vi "Linear_Flow_Ramp.vi"(2 "Debug Mode":bool, 3 "Elapsed Time (s)":dbl, 4 "State":enum16{"Edit", "Start", "Run", "End", "Idle"}(ring), 5 "Argument List In":string[](array[string])) -> (0 "Status Out":string, 1 "Argument List Out":string[](array[string]))   [LabVIEW 2011]
panel:
  in  "Flow to Ramp":u16(ring) items=["Flow1"]
  in  "Select":enum32{"Use Time/End Flow", "Use Rate"}(radio)
  in  "End Flow":dbl caption="End Flow\n(sccm)"
  in  "Total Time":dbl caption="Total Time (sec)"
  in  "Ramp Rate":dbl caption="Ramp Rate\n(sccm/sec)"
  in  "Start Flow":dbl caption="Start Flow\n(sccm)"
  in  "Gas":u16(ring)=5 items=["R_Al", "R_As_Liq", "R_AsH3", "R_Fe", "R_Ga", "R_H2", "R_In", "R_N_Dop", "R_N2", "R_P_Dop", "R_P_Liq", "R_PH3"]
  in  "Run":bool
  in  "Gas Source In":bool
  in  "H2 Flush":bool
  in  "Bubbler In":bool
  in  "H2 Dilute":bool
  in  "Cancel":bool
  in  "OK":bool
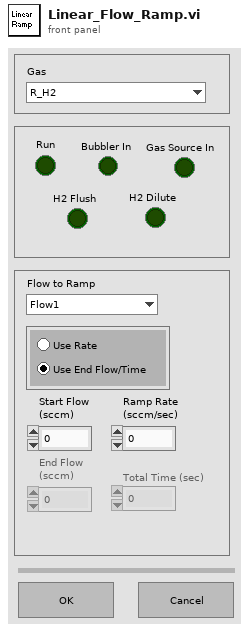
[diagram p1: front panel]
types:
  T1 = enum16{"Discrete", "Continuous", "Instantaneous"}
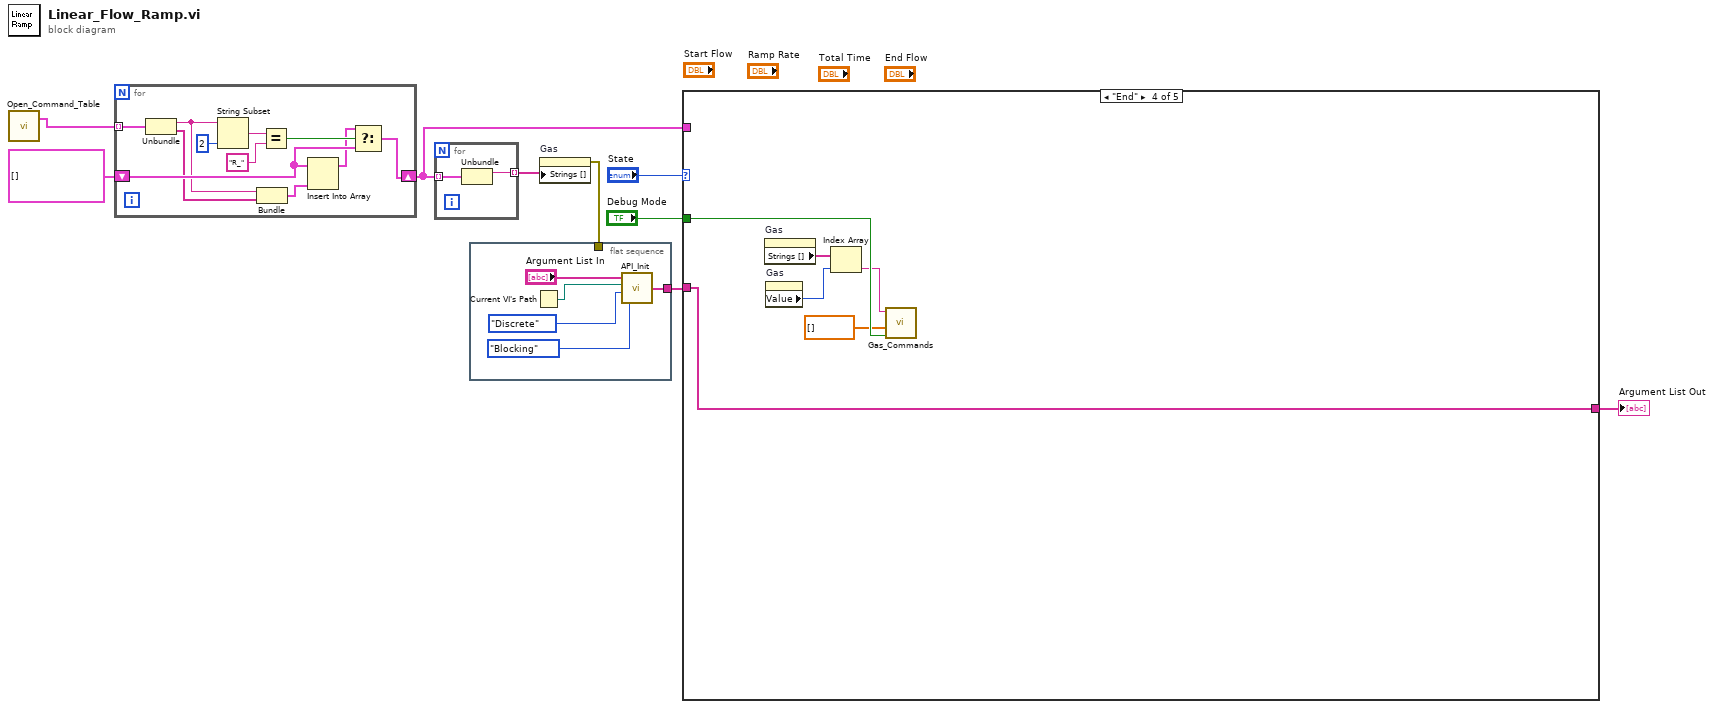
[diagram p0: block diagram]
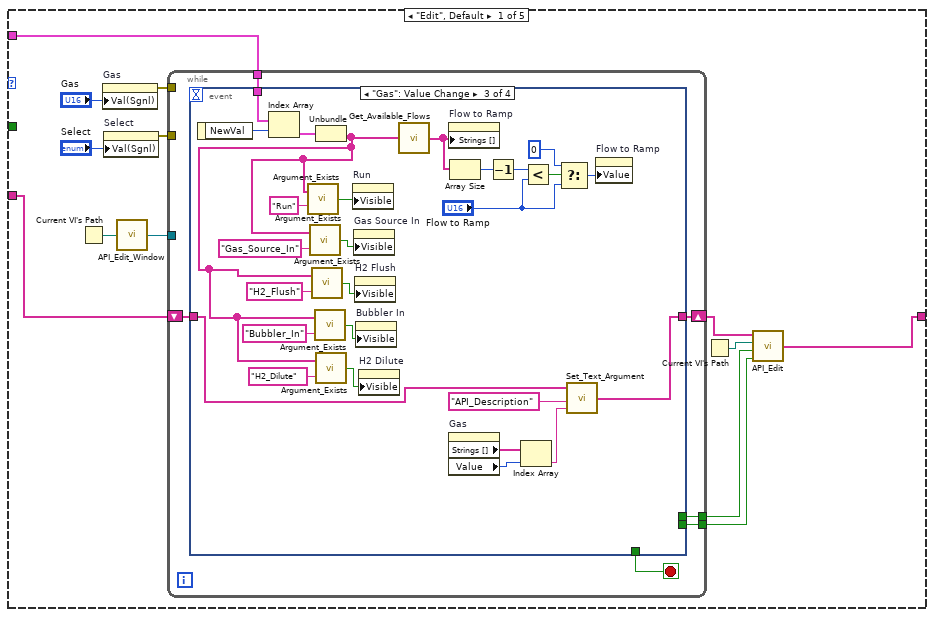
[diagram p2: hidden frame]
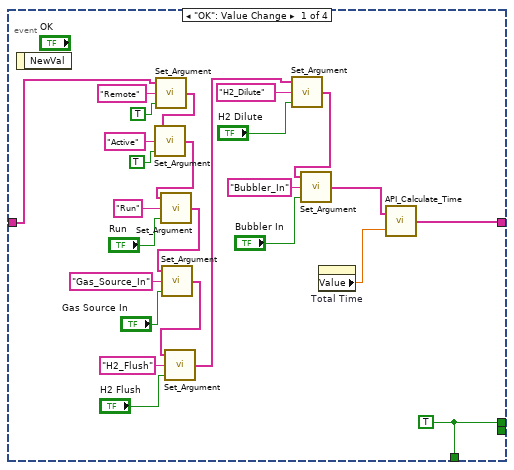
[diagram p3: hidden frame]
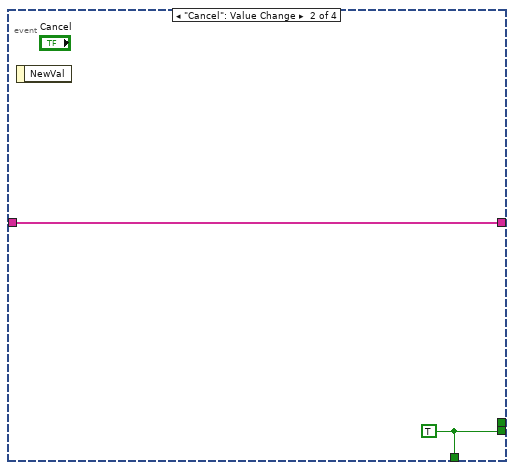
[diagram p4: hidden frame]
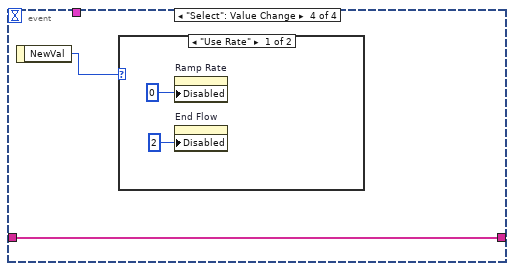
[diagram p5: hidden frame]
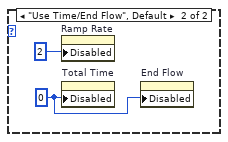
[diagram p6: hidden frame]
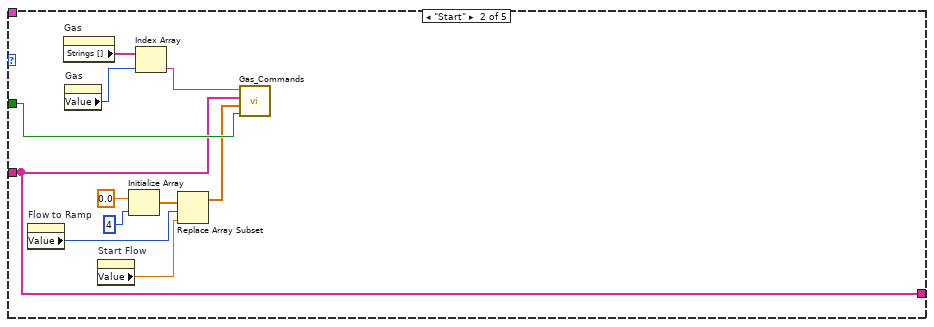
[diagram p7: hidden frame]
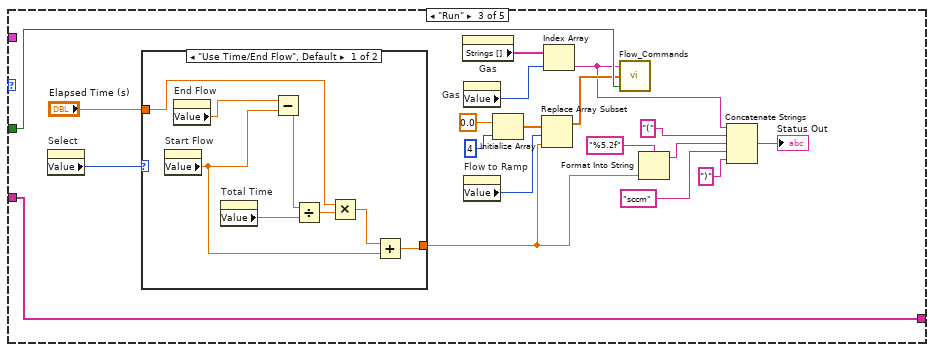
[diagram p8: hidden frame]
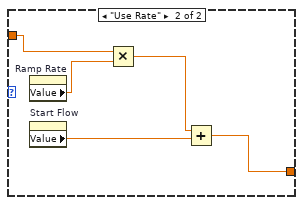
[diagram p9: hidden frame]
diagram:
  n1 = call "Open_Command_Table.vi"() -> ("Commands"=w3:cluster{string, string[]}[])  [unwired: 2 out]
  n2 = for {
    tunnel: w3 -> [w20] mode=indexing
    shift-right: [w15] -> w2
    shift-left: cluster{string, string[]}[] [] ("Commands") -> [w14]
    n3 = Unbundle(w20) -> (w12:string, w11:string[])
    n4 = String Subset(string=w12, length (rest)=2 ("length (rest)")) -> (substring=w18:string)  [unwired: 1 out]
    n5 = Bundle(w12, w11) -> (w10:cluster{string, string[]})  [unwired: 1 out]
    n6 = Equal?(x=w18, y="R_") -> (x = y?=w16:bool)
    n7 = Insert Into Array(array=w14, new element=w10) -> (w13:cluster{string, string[]}[])  [unwired: 1 in]
    n8 = Select(t=w13, s=w16, f=w14) -> (s? t:f=w15:cluster{string, string[]}[])
  }
  n9 = for {
    tunnel: w2 -> [w22] mode=indexing
    tunnel: [w21] -> w5 mode=indexing
    n10 = Unbundle(w22) -> (w21:string)  [unwired: 1 out]
  }
  n11 = flat-sequence {
    tunnel: [w27] -> w6
    tunnel: w1 -> [_]
    frame #0 {
      n12 = Current VI's Path() -> (path=w24:path)
      n13 = call "API_Init.vi"("API Option"=enum16{"None", "Blocking", "Wait for Input"}."Blocking", "API Mode"=T1."Discrete", "VI Path"=w24, "Argument List In"="Argument List In") -> ("Argument List Out"=w27:string[])
    }
  }
  n14 = property on="Gas" class="Ring (strict)"("Strings []"=w5) -> (error out=w1:errorcluster)  [unwired: 2 in, 1 out]
  n15 = case shown="\"End\"" "State" {
    tunnel: [w30 w110 w121 w153 w156] -> w8
    tunnel: w6 -> [w31 w110 w121 w153 w156]
    tunnel: "Debug Mode" -> [_ w117 w136 w155 _]
    tunnel: w2 -> [w34 _ _ _ _]
    frame "Edit", Default {
      n16 = Current VI's Path() -> (path=w36:path)
      n17 = property on="Gas" class="Ring (strict)"("Val(Sgnl)"="Gas") -> (error out=w32:errorcluster)  [unwired: 2 in, 1 out]
      n18 = property on="Select" class="RadioBtnsControl (strict)"("Val(Sgnl)"="Select") -> (error out=w28:errorcluster)  [unwired: 2 in, 1 out]
      n19 = call "API_Edit_Window.vi"("VI Path"=w36) -> ("VI Reference"=w35:refnum<vi>)
      n20 = while {
        tunnel: w34 -> [w45]
        tunnel: [w43] -> w38
        tunnel: [w42] -> w37
        tunnel: w35 -> [_]
        tunnel: w32 -> [_]
        shift-right: [w46] -> w39
        shift-left: w31 -> [w41]
        tunnel: w28 -> [_]
        stop <- w44 stop-if-true
        n21 = event shown="[2] \"Gas\": Value Change" {
          selector: _ -> [_ _ _ _]
          dyn-events: _ -> [_ _ _ _]
          timeout: _ -> [_ _ _ _]
          tunnel: w41 -> [w70 w73 w74 w101]
          tunnel: [w47 w73 w79 w101] -> w46
          tunnel: w45 -> [_ _ w100 _]
          tunnel: [w71 w72 _ _] -> w44
          tunnel: [w71 _ _ _] -> w43
          tunnel: [_ w72 _ _] -> w42
          event "OK": Value Change {
            w71 = TRUE
            n22 = event-data() -> ()  [unwired: 2 out]
            n23 = call "Set_Argument.vi"("Enable"=TRUE, "Argument"="Remote", "Argument List In"=w70) -> ("Argument List Out"=w51:string[])
            n24 = call "Set_Argument.vi"("Enable"=TRUE, "Argument"="Active", "Argument List In"=w51) -> ("Argument List Out"=w50:string[])
            n25 = call "Set_Argument.vi"("Enable"="Run", "Argument"="Run", "Argument List In"=w50) -> ("Argument List Out"=w65:string[])
            n26 = call "Set_Argument.vi"("Enable"="Gas Source In", "Argument"="Gas_Source_In", "Argument List In"=w65) -> ("Argument List Out"=w62:string[])
            n27 = call "Set_Argument.vi"("Enable"="H2 Flush", "Argument"="H2_Flush", "Argument List In"=w62) -> ("Argument List Out"=w59:string[])
            n28 = call "Set_Argument.vi"("Enable"="H2 Dilute", "Argument"="H2_Dilute", "Argument List In"=w59) -> ("Argument List Out"=w56:string[])
            n29 = call "Set_Argument.vi"("Enable"="Bubbler In", "Argument"="Bubbler_In", "Argument List In"=w56) -> ("Argument List Out"=w48:string[])
            n30 = property on="Total Time" class="DigNum (strict)"() -> ("Value"=w49:dbl)  [unwired: 2 in, 2 out]
            n31 = call "API_Calculate_Time.vi"("Time"=w49, "Argument List In"=w48) -> ("Argument List Out"=w47:string[])
          }
          event "Cancel": Value Change {
            w72 = TRUE
            n32 = event-data() -> ()  [unwired: 2 out]
          }
          event "Gas": Value Change {
            n33 = event-data() -> ("NewVal"=w88:u16)  [unwired: 1 out]
            n34 = Index Array(array=w100, index=w88) -> (element=w99:cluster{string, string[]})
            n35 = Unbundle(w99) -> (w83:string[])  [unwired: 1 out]
            n36 = call "Argument_Exists.vi"("Argument"="Run", "Argument List"=w83) -> ("Argument Exists"=w97:bool)
            n37 = call "Argument_Exists.vi"("Argument"="Gas_Source_In", "Argument List"=w83) -> ("Argument Exists"=w93:bool)
            n38 = call "Argument_Exists.vi"("Argument"="H2_Flush", "Argument List"=w83) -> ("Argument Exists"=w94:bool)
            n39 = call "Argument_Exists.vi"("Argument"="Bubbler_In", "Argument List"=w83) -> ("Argument Exists"=w91:bool)
            n40 = call "Argument_Exists.vi"("Argument"="H2_Dilute", "Argument List"=w83) -> ("Argument Exists"=w89:bool)
            n41 = property on="Run" class="Bool (strict)"("Visible"=w97) -> ()  [unwired: 2 in, 2 out]
            n42 = property on="Gas Source In" class="Bool (strict)"("Visible"=w93) -> ()  [unwired: 2 in, 2 out]
            n43 = property on="H2 Flush" class="Bool (strict)"("Visible"=w94) -> ()  [unwired: 2 in, 2 out]
            n44 = property on="Bubbler In" class="Bool (strict)"("Visible"=w91) -> ()  [unwired: 2 in, 2 out]
            n45 = property on="H2 Dilute" class="Bool (strict)"("Visible"=w89) -> ()  [unwired: 2 in, 2 out]
            n46 = call "Get_Available_Flows.vi"("Argument List"=w83) -> ("Available Flows"=w81:string[])
            n47 = property on="Flow to Ramp" class="Ring (strict)"("Strings []"=w81) -> ()  [unwired: 2 in, 2 out]
            n48 = property on="Gas" class="Ring (strict)"() -> ("Strings []"=w78:string[], "Value"=w77:u16)  [unwired: 2 in, 2 out]
            n49 = Array Size(array=w81) -> (size(s)=w87:i32)
            n50 = Decrement(x=w87) -> (x-1=w85:i32)
            n51 = Index Array(array=w78, index=w77) -> (element=w76:string)
            n52 = Less?(x=w85, y="Flow to Ramp") -> (x < y?=w86:bool)
            n53 = Select(t=u16 0, s=w86, f="Flow to Ramp") -> (s? t:f=w75:u16)
            n54 = call "Set_Text_Argument.vi"("Text"=w76, "Argument"="API_Description", "Argument List In"=w74) -> ("Argument List Out"=w79:string[])
            n55 = property on="Flow to Ramp" class="Ring (strict)"("Value"=w75) -> ()  [unwired: 2 in, 2 out]
          }
          event "Select": Value Change {
            n56 = event-data() -> ("NewVal"=w102:enum32{"Use Time/End Flow", "Use Rate"})  [unwired: 1 out]
            n57 = case shown="\"Use Rate\"" w102 {
              frame "Use Rate" {
                n58 = property on="Ramp Rate" class="DigNum (strict)"("Disabled"=u8 0) -> ()  [unwired: 2 in, 2 out]
                n59 = property on="End Flow" class="DigNum (strict)"("Disabled"=u8 2) -> ()  [unwired: 2 in, 2 out]
              }
              frame "Use Time/End Flow", Default {
                w105 = u8 0 ("Disabled")
                n60 = property on="Ramp Rate" class="DigNum (strict)"("Disabled"=u8 2) -> ()  [unwired: 2 in, 2 out]
                n61 = property on="Total Time" class="DigNum (strict)"("Disabled"=w105) -> ()  [unwired: 2 in, 2 out]
                n62 = property on="End Flow" class="DigNum (strict)"("Disabled"=w105) -> ()  [unwired: 2 in, 2 out]
              }
            }
          }
        }
      }
      n63 = Current VI's Path() -> (path=w40:path)
      n64 = call "API_Edit.vi"("Cancel"=w37, "OK"=w38, "VI Path"=w40, "Argument List In"=w39) -> ("Argument List Out"=w30:string[])
    }
    frame "Start" {
      n65 = property on="Flow to Ramp" class="Ring (strict)"() -> ("Value"=w114:u16)  [unwired: 2 in, 2 out]
      n66 = property on="Gas" class="Ring (strict)"() -> ("Strings []"=w109:string[])  [unwired: 2 in, 2 out]
      n67 = property on="Gas" class="Ring (strict)"() -> ("Value"=w108:u16)  [unwired: 2 in, 2 out]
      n68 = property on="Start Flow" class="DigNum (strict)"() -> ("Value"=w112:dbl)  [unwired: 2 in, 2 out]
      n69 = Initialize Array(0.0 ("element"), 4 ("dimension size")) -> (w113:dbl[])
      n70 = Index Array(array=w109, index=w108) -> (element=w107:string)
      n71 = Replace Array Subset(array=w113, new element=w112, index=w114) -> (w111:dbl[])
      n72 = call "Gas_Commands.vi"("Debug Mode"=w117, "Flow Array"=w111, "Argument List"=w110, "Command"=w107) -> ()  [unwired: 1 out]
    }
    frame "Run" {
      n73 = property on="Select" class="RadioBtnsControl (strict)"() -> ("Value"=w122:enum32{"Use Time/End Flow", "Use Rate"})  [unwired: 2 in, 2 out]
      n74 = case shown="\"Use Time/End Flow\", Default" w122 {
        tunnel: "Elapsed Time (s)" -> [w143 w149]
        tunnel: [w137 w145] -> w126
        frame "Use Time/End Flow", Default {
          n75 = property on="Start Flow" class="DigNum (strict)"() -> ("Value"=w139:dbl)  [unwired: 2 in, 2 out]
          n76 = property on="End Flow" class="DigNum (strict)"() -> ("Value"=w141:dbl)  [unwired: 2 in, 2 out]
          n77 = property on="Total Time" class="DigNum (strict)"() -> ("Value"=w142:dbl)  [unwired: 2 in, 2 out]
          n78 = Subtract(x=w141, y=w139) -> (x-y=w140:dbl)
          n79 = Divide(x=w140, y=w142) -> (x/y=w144:dbl)
          n80 = Multiply(x=w143, y=w144) -> (x*y=w138:dbl)
          n81 = Add(x=w138, y=w139) -> (x+y=w137:dbl)
        }
        frame "Use Rate" {
          n82 = property on="Ramp Rate" class="DigNum (strict)"() -> ("Value"=w148:dbl)  [unwired: 2 in, 2 out]
          n83 = property on="Start Flow" class="DigNum (strict)"() -> ("Value"=w146:dbl)  [unwired: 2 in, 2 out]
          n84 = Multiply(x=w149, y=w148) -> (x*y=w147:dbl)
          n85 = Add(x=w147, y=w146) -> (x+y=w145:dbl)
        }
      }
      n86 = property on="Gas" class="Ring (strict)"() -> ("Strings []"=w119:string[])  [unwired: 2 in, 2 out]
      n87 = property on="Gas" class="Ring (strict)"() -> ("Value"=w120:u16)  [unwired: 2 in, 2 out]
      n88 = property on="Flow to Ramp" class="Ring (strict)"() -> ("Value"=w131:u16)  [unwired: 2 in, 2 out]
      n89 = Initialize Array(0.0 ("element"), 4 ("dimension size")) -> (w132:dbl[])
      n90 = Replace Array Subset(array=w132, new element=w126, index=w131) -> (w130:dbl[])
      n91 = Index Array(array=w119, index=w120) -> (element=w118:string)
      n92 = call "Flow_Commands.vi"("Debug Mode"=w136, "Flow Array"=w130, "Command"=w118) -> ()  [unwired: 1 out]
      n93 = Format Into String(format string="%5.2f", w126) -> (resulting string=w125:string)  [unwired: 2 in, 1 out]
      n94 = Concatenate Strings(w118, "(" ("string"), w125, "sccm" ("string"), ")" ("string")) -> (→"Status Out":string)
    }
    frame "End" {
      n95 = property on="Gas" class="Ring (strict)"() -> ("Strings []"=w151:string[])  [unwired: 2 in, 2 out]
      n96 = property on="Gas" class="Ring (strict)"() -> ("Value"=w152:u16)  [unwired: 2 in, 2 out]
      n97 = Index Array(array=w151, index=w152) -> (element=w150:string)
      n98 = call "Gas_Commands.vi"("Debug Mode"=w155, "Flow Array"=dbl[] [], "Command"=w150) -> ()  [unwired: 1 in, 1 out]
    }
    frame "Idle" {
    }
  }
  "Argument List Out" <- w8
